vi "Load Packed Libraries.vi"(8 "error in (no error)":errorcluster, 10 "packed library names":string[](array[string]), 11 "Component Loader in":refnum<class "Component Loader.lvclass">) -> (0 "error out":errorcluster, 2 "objects":refnum<class>[](array[class]), 3 "Component Loader out":refnum<class "Component Loader.lvclass">)   [LabVIEW 2017, in "DSF Core.lvlib" / "Component Loader.lvclass"]
uses:
  Component Loader.lvclass
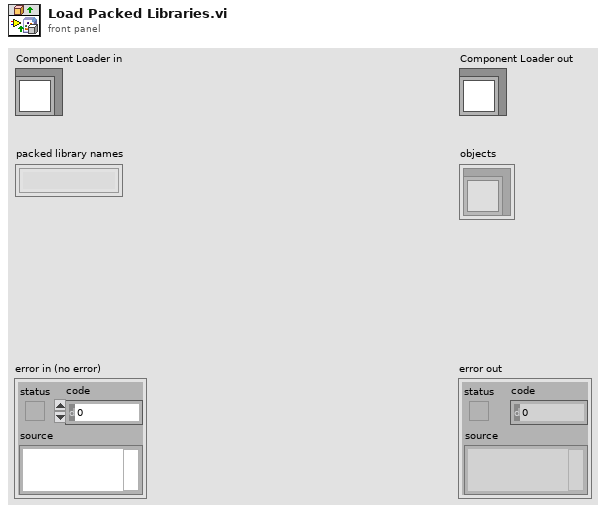
[diagram p1: front panel]
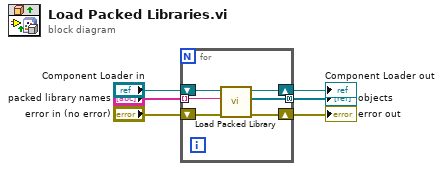
[diagram p0: block diagram]
diagram:
  n1 = for {
    shift-right: [w9] -> w3
    shift-left: "Component Loader in" -> [w12]
    shift-right: [w10] -> w2
    shift-left: "error in (no error)" -> [w11]
    tunnel: [w8] -> w4 mode=concatenating
    tunnel: "packed library names" -> [w7] mode=indexing
    n2 = call "Load Packed Library.vi"("error in (no error)"=w11, "packed library name"=w7, "Component Loader in"=w12) -> ("error out"=w10:errorcluster, "objects"=w8:refnum<class>[], "Component Loader out"=w9:refnum<class "Component Loader.lvclass">)  [unwired: 6 in]
  }
  "error out" <- w2
  "Component Loader out" <- w3
  "objects" <- w4
